vi "poly_sub(m)_filter.vi"(8 "error in (no error)":errorcluster, 9 "f":i32=50 caption="base frequency (50Hz)", 10 "N":i32=3 caption="N of harmonics to remove (3)", 11 "array of xwavs in":T1[](array[typedef])) -> (0 "error out":errorcluster, 3 "array of xwavs out":T1[](array[typedef]))   [LabVIEW 2015]
uses:
  xwave/xwav.ctl
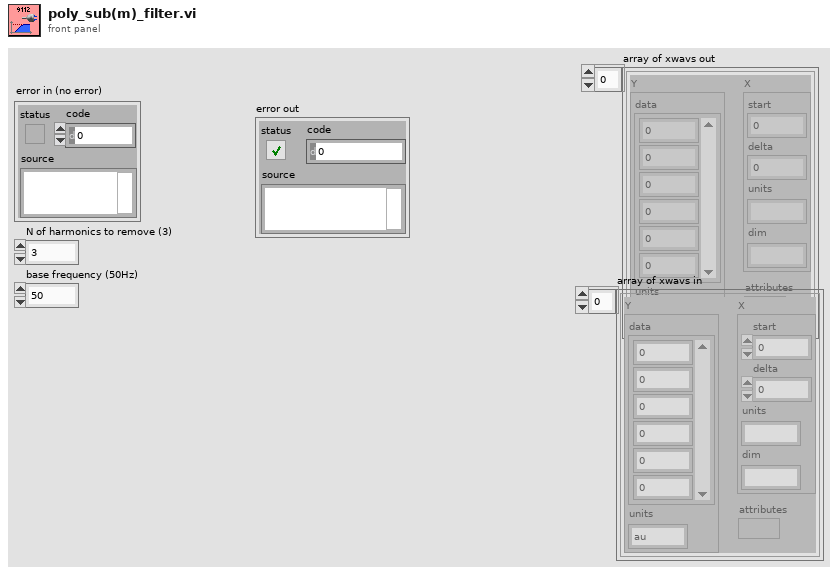
[diagram p1: front panel]
types:
  T1 = typedef "xwav.ctl" = cluster{"attributes":variant, "X":cluster{"start":dbl, "delta":dbl, "units":string, "dim":string}, "Y":cluster{"data":dbl[], "units":string}}
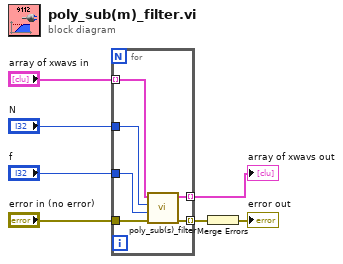
[diagram p0: block diagram]
diagram:
  n1 = for {
    tunnel: "N" -> [w13]
    tunnel: "f" -> [w12]
    tunnel: "error in (no error)" -> [w11]
    tunnel: [w10] -> w2 mode=indexing
    tunnel: [w9] -> w4 mode=indexing
    tunnel: "array of xwavs in" -> [w8] mode=indexing
    n2 = call "poly_sub(s)_filter.vi"("error in (no error)"=w11, "f"=w12, "N"=w13, "xwave in"=w8) -> ("error out"=w9:errorcluster, "xwave out"=w10:T1)  [unwired: 6 in]
  }
  "array of xwavs out" <- w2
  n3 = Merge Errors(w4) -> (→"error out":errorcluster)
